vi "mxwScript_Cmnd2Str_deuniquifyObject.vi"(8 "error in (no error)":errorcluster, 11 "data":variant) -> (0 "error out":errorcluster, 3 "outputString":string)   [LabVIEW 2020]
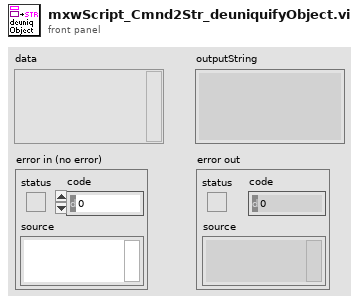
[diagram p1: front panel]
types:
  T1 = cluster{"controlName":string, "finalControlName":string, "templateIndex":i32}
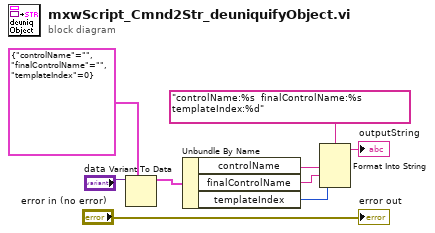
[diagram p0: block diagram]
diagram:
  n1 = Variant To Data(type=T1 {"controlName"="", "finalControlName"="", "templateIndex"=0}, Variant="data") -> (data=w8:T1)  [unwired: 1 in, 1 out]
  n2 = Unbundle By Name(w8) -> ("controlName"=w4:string, "finalControlName"=w1:string, "templateIndex"=w2:i32)
  n3 = Format Into String(format string="controlName:%s  finalControlName:%s  templateIndex:%d", w4, w1, w2) -> (resulting string=→"outputString":string)  [unwired: 2 in, 1 out]
  "error out" <- "error in (no error)"
